vi "control_panel.vi"() -> ()   [LabVIEW 2022 SP3]
uses:
  led_indicator.ctl
  <vilib>/Utility/miscctls.llb/LVPositionTypeDef.ctl
  global_variable_STOP.vi
panel:
  out "DET_VENT_OX":bool
  out "DET_VENT_FU":bool
  out "DET_PRESS_OX":bool
  out "DET_PRESS_FU":bool
  out "DET_MAIN_OX":bool
  out "DET_MAIN_FU":bool
  out "DET_FILL_OX":bool
  out "DET_FILL_FU":bool
  out "DET_PURGE_OX":bool
  out "DET_PURGE_FU":bool
  out "DET_EMATCH":bool
  out "FBK_MBV":T1
  in  "ACTI_VENT_FU":bool
  in  "ACTI_VENT_OX":bool
  out "LOG_TRIG_STATUS":dbl
  in  "LOG_TRIG_ON":bool
  in  "ACT_WINCH_ON":bool
  in  "ACT_WINCH_DIR":bool
  in  "ACT_MAIN_FU":bool
  out "FBK_MAIN_FU":bool
  in  "ACT_PRESS_FU":bool
  in  "ACT_FILL_OX":bool
  in  "ACT_PRESS_OX":bool
  in  "ACT_MBV":bool
  in  "ACT_MAIN_OX":bool
  in  "ACT_FILL_FU":bool
  in  "ACT_EMATCH":bool
  in  "ACT_PURGE_OX":bool
  in  "ACT_PURGE_FU":bool
  out "FBK_MAIN_OX":T1
  out "FBK_PRESS_FU":T1
  out "FBK_PRESS_OX":T1
  out "FBK_VENT_FU":T1
  out "FBK_VENT_OX":T1
  out "FBK_FILL_OX":T1
  out "FBK_FILL_FU":T1
  out "FBK_PURGE_OX":T1
  out "FBK_PURGE_FU":T1
  in  "ACT_SIREN":bool
  # "Command"
  # "Feedback"
  # "Command"
  # "Feedback"
  # "Command"
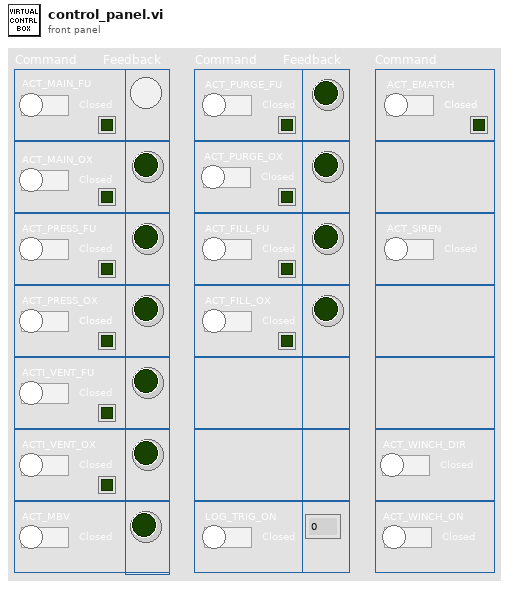
[diagram p1: front panel]
types:
  T1 = typedef "led_indicator.ctl" = bool
  T2 = typedef "LVPositionTypeDef.ctl" = cluster{"Left":i32, "Top":i32}
  T3 = typedef "Semaphore RefNum" = refnum<k1>
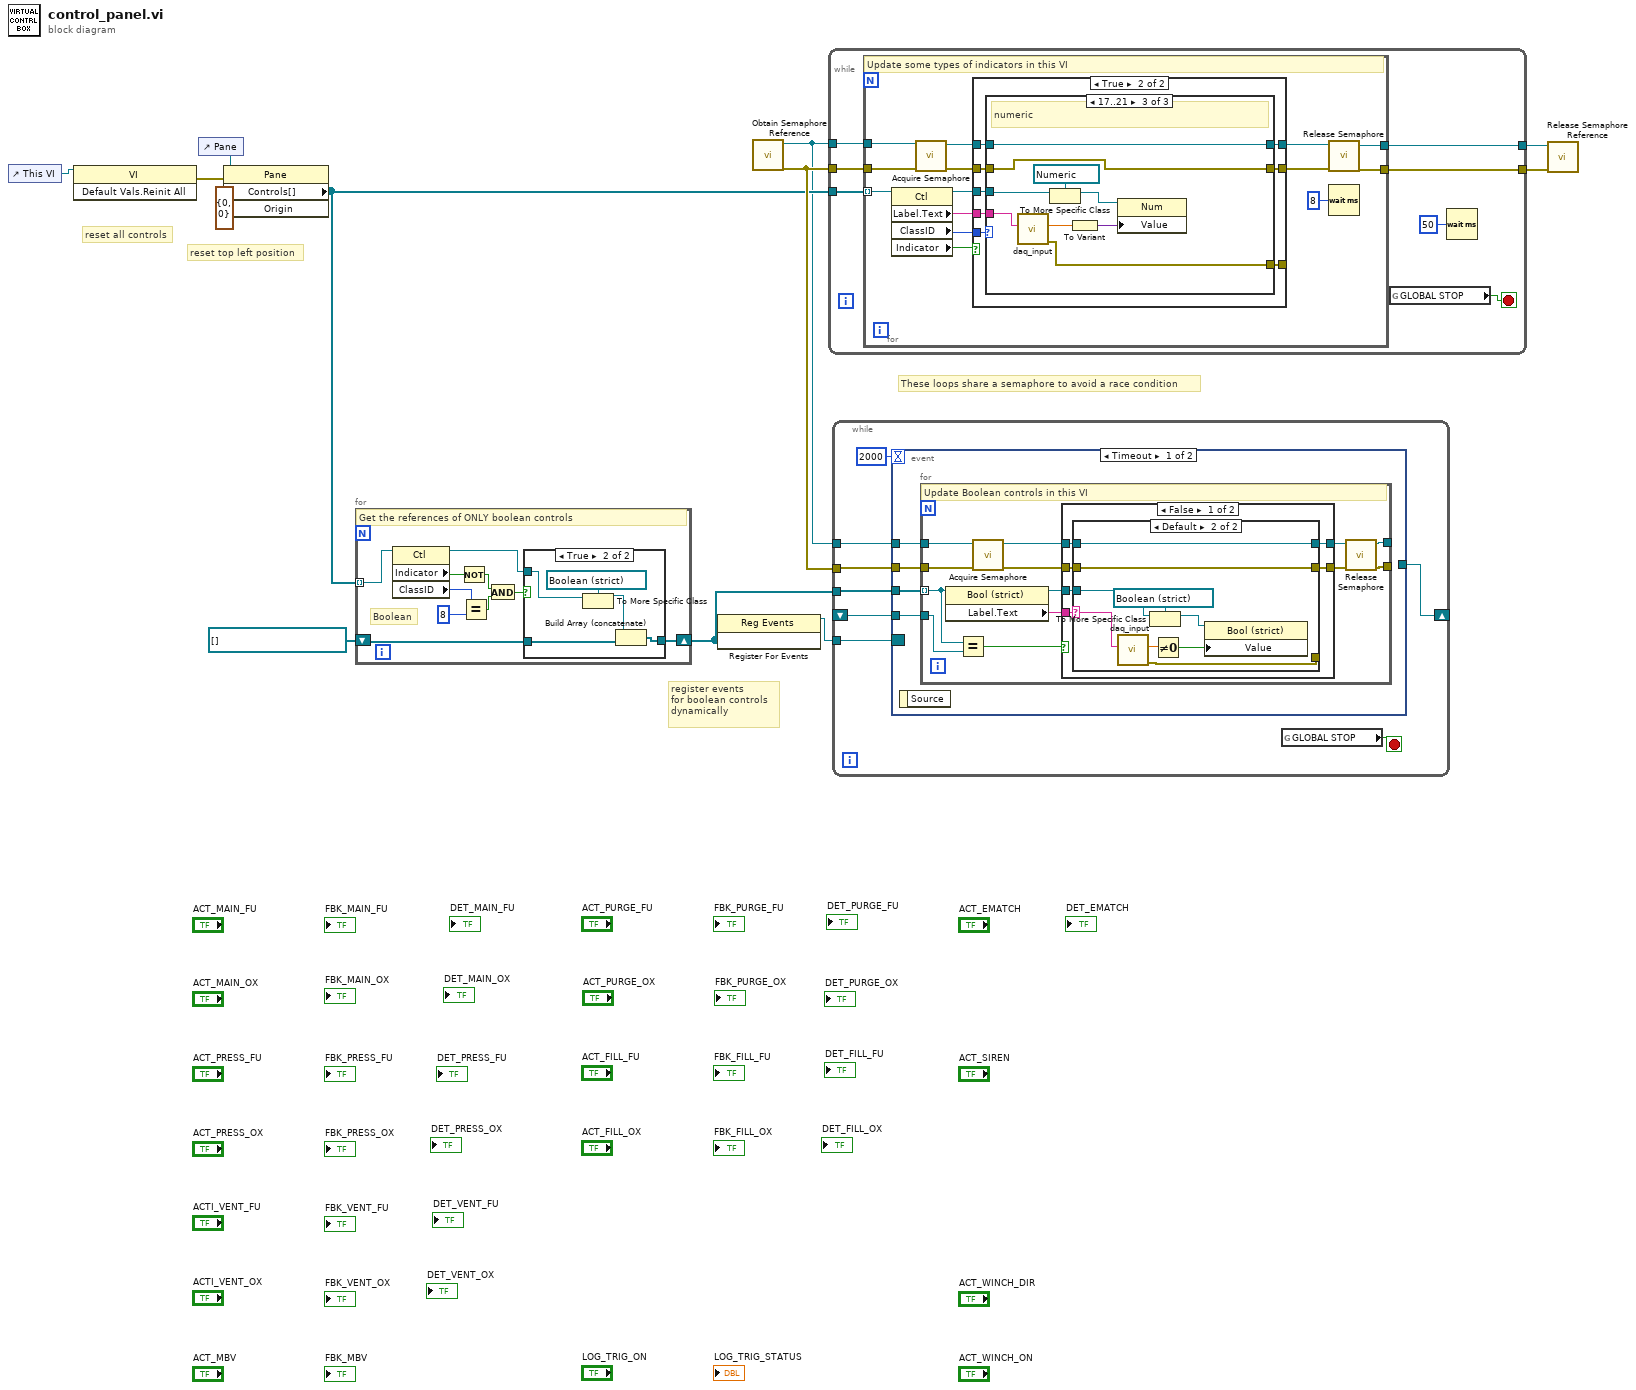
[diagram p0: block diagram]
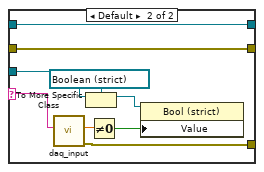
[diagram p5: hidden frame]
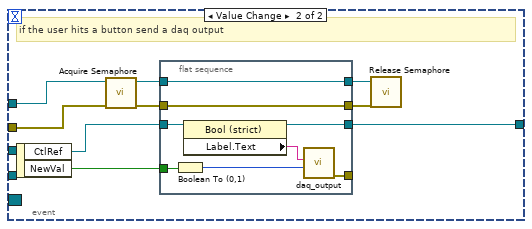
[diagram p8: hidden frame]
diagram:
  # "reset top left position"
  # "reset all controls"
  # "These loops share a semaphore to avoid a race condition"
  # "register events\nfor boolean controls\ndynamically"
  n1 = control-ref of="This VI"() -> (w11:refnum<vi>)
  n2 = invoke class="VI" method="Default Vals.Reinit All"(reference=w11) -> (error out=w10:errorcluster)  [unwired: 2 in, 2 out]
  n3 = control-ref of="Pane"() -> (w12:refnum<vi>)
  n4 = property class="Pane"(reference=w12, error in=w10, "Origin"=T2 {"Left"=0, "Top"=0} ("Position")) -> ("Controls[]"=w3:refnum<vi>[])  [unwired: 2 out]
  n5 = for {
    tunnel: w3 -> [w20] mode=indexing
    shift-right: [w14] -> w1
    shift-left: refnum<vi>[] [] -> [w13]
    # "Boolean"
    # "Get the references of ONLY boolean controls"
    n6 = property class="Ctl"(reference=w20) -> (reference out=w15:refnum<vi>, "Indicator"=w16:bool, "ClassID"=w22:u32)  [unwired: 1 in, 1 out]
    n7 = Not(x=w16) -> (.not. x?=w17:bool)
    n8 = Equal?(x=w22, y=u32 8) -> (x = y?=w18:bool)
    n9 = And(x=w17, y=w18) -> (x .and. y?=w19:bool)
    n10 = case shown="True" w19 {
      tunnel: w15 -> [_ w27]
      tunnel: [w23 w26] -> w14
      tunnel: w13 -> [w23 w24]
      frame False {
      }
      frame True {
        n11 = To More Specific Class(target class=refnum<vi> refnum ("Bool Refnum"), reference=w27) -> (specific class reference=w25:refnum<vi>)  [unwired: 1 in, 1 out]
        n12 = Build Array (concatenate)(w25, w24) -> (w26:refnum<vi>[])
      }
    }
  }
  n13 = register-events(w1) -> (reference out=w9:refnum<event-registration>)  [unwired: 2 in, 1 out]
  n14 = call <vilib>:"Obtain Semaphore Reference.vi"() -> ("error out"=w7:errorcluster, "semaphore"=w2:T3)  [unwired: 5 in, 1 out]
  n15 = while {
    tunnel: w3 -> [w35]
    tunnel: w2 -> [w34]
    tunnel: w7 -> [w33]
    tunnel: [w31] -> w6
    tunnel: [w30] -> w5
    stop <- w32 stop-if-true
    n16 = for {
      tunnel: w35 -> [w47] mode=indexing
      tunnel: w34 -> [w42]
      tunnel: w33 -> [w41]
      tunnel: [w40] -> w31
      tunnel: [w39] -> w30
      # "Update some types of indicators in this VI"
      n17 = property class="Ctl"(reference=w47) -> (reference out=w48:refnum<vi>, "Label.Text"=w49:string, "ClassID"=w37:u32, "Indicator"=w36:bool)  [unwired: 1 in, 1 out]
      n18 = call <vilib>:"Acquire Semaphore.vi"("error in (no error)"=w41, "semaphore"=w42) -> ("error out"=w44:errorcluster, "semaphore out"=w46:T3)  [unwired: 3 in, 1 out]
      n19 = case shown="True" w36 {
        tunnel: w49 -> [_ w59]
        tunnel: w48 -> [_ w58]
        tunnel: w46 -> [w51 w57]
        tunnel: [w51 w56] -> w45
        tunnel: w44 -> [w50 w55]
        tunnel: [w50 w54] -> w43
        tunnel: w37 -> [_ w53]
        tunnel: [_ w52] -> _
        frame False {
        }
        frame True {
          n20 = case shown="17..21" w53 {
            tunnel: w59 -> [_ w67 w83]
            tunnel: w58 -> [_ w68 w84]
            tunnel: [w61 w64 w81] -> w56
            tunnel: w57 -> [w61 w66 w81]
            tunnel: [w60 w63 w82] -> w54
            tunnel: w55 -> [w60 w65 w82]
            tunnel: [_ w62 w80] -> w52
            frame Default {
              # "do nothing"
              # "other"
            }
            frame 8 {
              # "boolean"
              n21 = case shown="\"LOG_TRIG_ON\"" w67 {
                selector: w67 -> [_ w74]
                tunnel: w68 -> [_ w75]
                tunnel: [w70 w72] -> w64
                tunnel: w66 -> [w70 w72]
                tunnel: [w69 w73] -> w63
                tunnel: w65 -> [w69 w73]
                tunnel: [_ w71] -> w62
                frame "LOG_TRIG_ON" {
                  # "special case, do not update"
                }
                frame Default {
                  n22 = call "daq_input.vi"("channel"=w74) -> ("error out"=w71:errorcluster, "value"=w79:dbl)  [unwired: 9 in]
                  n23 = To More Specific Class(target class=refnum<vi> refnum ("Bool Refnum"), reference=w75) -> (specific class reference=w77:refnum<vi>)  [unwired: 1 in, 1 out]
                  n24 = Not Equal To 0?(x=w79) -> (x != 0?=w76:bool)
                  n25 = property on="Property Node" class="Bool (strict)"(reference=w77, "Value"=w76) -> ()  [unwired: 1 in, 2 out]
                }
              }
            }
            frame 17..21 {
              # "numeric"
              n26 = call "daq_input.vi"("channel"=w83) -> ("error out"=w80:errorcluster, "value"=w85:dbl)  [unwired: 9 in]
              n27 = To More Specific Class(target class=refnum<vi> refnum ("Num Refnum"), reference=w84) -> (specific class reference=w88:refnum<vi>)  [unwired: 1 in, 1 out]
              n28 = To Variant(anything=w85) -> (Variant=w87:variant)
              n29 = property on="Property Node" class="Num"(reference=w88, "Value"=w87) -> ()  [unwired: 1 in, 2 out]
            }
          }
        }
      }
      n30 = call <vilib>:"Release Semaphore.vi"("error in (no error)"=w43, "semaphore"=w45) -> ("error out"=w39:errorcluster, "semaphore out"=w40:T3)  [unwired: 4 in]
      n31 = Wait (ms)(milliseconds to wait=u32 8) -> ()  [unwired: 1 out]
    }
    n32 = global read "global_variable_STOP.vi" "GLOBAL STOP"() -> (w32:bool)
    n33 = Wait (ms)(milliseconds to wait=u32 50) -> ()  [unwired: 1 out]
  }
  n34 = while {
    tunnel: w9 -> [w96]
    tunnel: w7 -> [w92]
    tunnel: w1 -> [w91]
    tunnel: w2 -> [w93]
    shift-right: [w90] -> _
    shift-left: _ -> [w89]
    stop <- w95 stop-if-true
    n35 = event shown="[0] Timeout" {
      selector: w96 -> [_ _]
      dyn-events: _ -> [_ _]
      timeout: 2000 -> [_ _]
      tunnel: w93 -> [w100 w135]
      tunnel: w92 -> [w99 w134]
      tunnel: w91 -> [w98 _]
      tunnel: [_ w133] -> w90
      tunnel: w89 -> [w97 _]
      event Timeout {
        n36 = event-data() -> ()  [unwired: 1 in, 1 out]
        n37 = for {
          tunnel: [w107] -> _
          tunnel: [w106] -> _
          tunnel: w100 -> [w105]
          tunnel: w99 -> [w104]
          tunnel: w98 -> [w103] mode=indexing
          tunnel: w97 -> [w102]
          # "Update Boolean controls in this VI"
          n38 = property class="Bool (strict)"(reference=w103) -> (reference out=w112:refnum<vi>, "Label.Text"=w113:string)  [unwired: 1 in, 1 out]
          n39 = Equal?(x=w103, y=w102) -> (x = y?=w101:bool)
          n40 = call <vilib>:"Acquire Semaphore.vi"("error in (no error)"=w104, "semaphore"=w105) -> ("error out"=w109:errorcluster, "semaphore out"=w111:T3)  [unwired: 3 in, 1 out]
          n41 = case shown="False" w101 {
            tunnel: w113 -> [w119 _]
            tunnel: w112 -> [w118 _]
            tunnel: w111 -> [w117 w132]
            tunnel: [w116 w132] -> w110
            tunnel: w109 -> [w115 w131]
            tunnel: [w114 w131] -> w108
            frame False {
              n42 = case shown="Default" w119 {
                selector: w119 -> [_ w125]
                tunnel: w118 -> [_ w126]
                tunnel: [w121 w123] -> w116
                tunnel: w117 -> [w121 w123]
                tunnel: [w120 w124] -> w114
                tunnel: w115 -> [w120 w124]
                tunnel: [_ w122] -> _
                frame "////LOG_TRIG_ON" {
                  # "special case, do not update"
                }
                frame Default {
                  n43 = call "daq_input.vi"("channel"=w125) -> ("error out"=w122:errorcluster, "value"=w130:dbl)  [unwired: 9 in]
                  n44 = To More Specific Class(target class=refnum<vi> refnum ("Bool Refnum"), reference=w126) -> (specific class reference=w128:refnum<vi>)  [unwired: 1 in, 1 out]
                  n45 = Not Equal To 0?(x=w130) -> (x != 0?=w127:bool)
                  n46 = property on="Property Node" class="Bool (strict)"(reference=w128, "Value"=w127) -> ()  [unwired: 1 in, 2 out]
                }
              }
            }
            frame True {
            }
          }
          n47 = call <vilib>:"Release Semaphore.vi"("error in (no error)"=w108, "semaphore"=w110) -> ("error out"=w106:errorcluster, "semaphore out"=w107:T3)  [unwired: 4 in]
        }
      }
      event Value Change {
        # "if the user hits a button send a daq output"
        n48 = event-data() -> ("CtlRef"=w141:refnum<vi>, "NewVal"=w140:bool)  [unwired: 1 in]
        n49 = call <vilib>:"Acquire Semaphore.vi"("error in (no error)"=w134, "semaphore"=w135) -> ("error out"=w137:errorcluster, "semaphore out"=w139:T3)  [unwired: 3 in, 1 out]
        n50 = flat-sequence {
          tunnel: w141 -> [w149]
          tunnel: w140 -> [w147]
          tunnel: [w145] -> w138
          tunnel: w139 -> [w145]
          tunnel: [w144] -> w136
          tunnel: w137 -> [w144]
          tunnel: [w143] -> _
          tunnel: [w142] -> w133
          frame #0 {
            n51 = Boolean To (0,1)(Boolean=w147) -> (0, 1=w146:i16)
            n52 = property class="Bool (strict)"(reference=w149) -> (reference out=w142:refnum<vi>, "Label.Text"=w148:string)  [unwired: 1 in, 1 out]
            n53 = call "daq_output.vi"("value"=w146, "channel"=w148) -> ("error out"=w143:errorcluster)  [unwired: 9 in]
          }
        }
        n54 = call <vilib>:"Release Semaphore.vi"("error in (no error)"=w136, "semaphore"=w138) -> ()  [unwired: 4 in, 2 out]
      }
    }
    n55 = global read "global_variable_STOP.vi" "GLOBAL STOP"() -> (w95:bool)
  }
  n56 = call <vilib>:"Release Semaphore Reference.vi"("error in (no error)"=w5, "semaphore"=w6) -> ()  [unwired: 8 in, 2 out]
